vi "niFPGA Fractional Interval.vi"   [LabVIEW 2017]
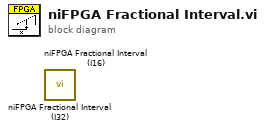
[diagram p0: block diagram]
diagram:
  n1 = call <vilib>:"niFPGA Fractional Interval (I32).vi"() -> ()  [unwired: 11 in, 1 out]
  n2 = call <vilib>:"niFPGA Fractional Interval (I16).vi"() -> ()  [unwired: 11 in, 1 out]
